vi "dryRunTest.vi"() -> ()   [LabVIEW 2015]
uses:
  GlobalPath.vi
  GlobalData.vi
  GlobalVi.vi
panel:
  in  "Done?":bool
  in  "Open Gauge Program 2":bool
  in  "Full or empty?":bool
  in  "Done?":bool
  in  "Open Gauge Program":bool
  in  "c-ccd 14":bool caption="Stiffback surface measurement with gauge system"
  in  "c-ccd 13":bool caption="Micrometer measurement of the distance between the reference plates \nand the stiffback plates along the perimeter"
  in  "c-ccd 12":bool caption="Position the weights on the stiffback"
  in  "c-ccd 11":bool caption="Release the stiffback from the movement arch"
  in  "c-ccd 10":bool caption="Lower the stiffback on the reference plates"
  in  "c-ccd 9":bool caption="Move the stiffback over the reference plates"
  in  "c-ccd 8":bool caption="Rotate the stiffback upside down"
  in  "c-ccd 7":bool caption="Check cleanness of the 20 stiffback supports"
  in  "c-ccd 6":bool caption="Mount the 2 stiffback-alignment pins on the reference plates"
  in  "c-ccd 5":bool caption="Position the honeycomb on the PCBs"
  in  "c-ccd 4":bool caption="Position the 4 internal frames in correspondence to the PCB-to-PCB junction"
  in  "c-ccd 3":bool caption="Position the 6 extrenal frames using 12 PTFE pins"
  # "Dry run preparation"
  # "Dry run empty/full"
  # "(True if full)"
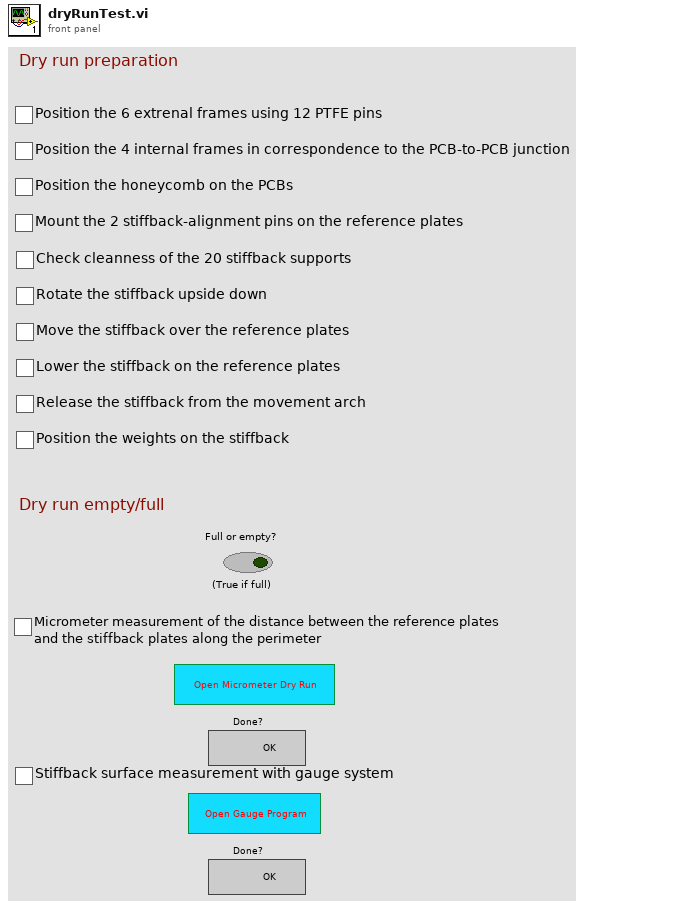
[diagram p1: front panel]
types:
  T1 = enum32{"Bad", "Idle", "Run top level", "Running"}
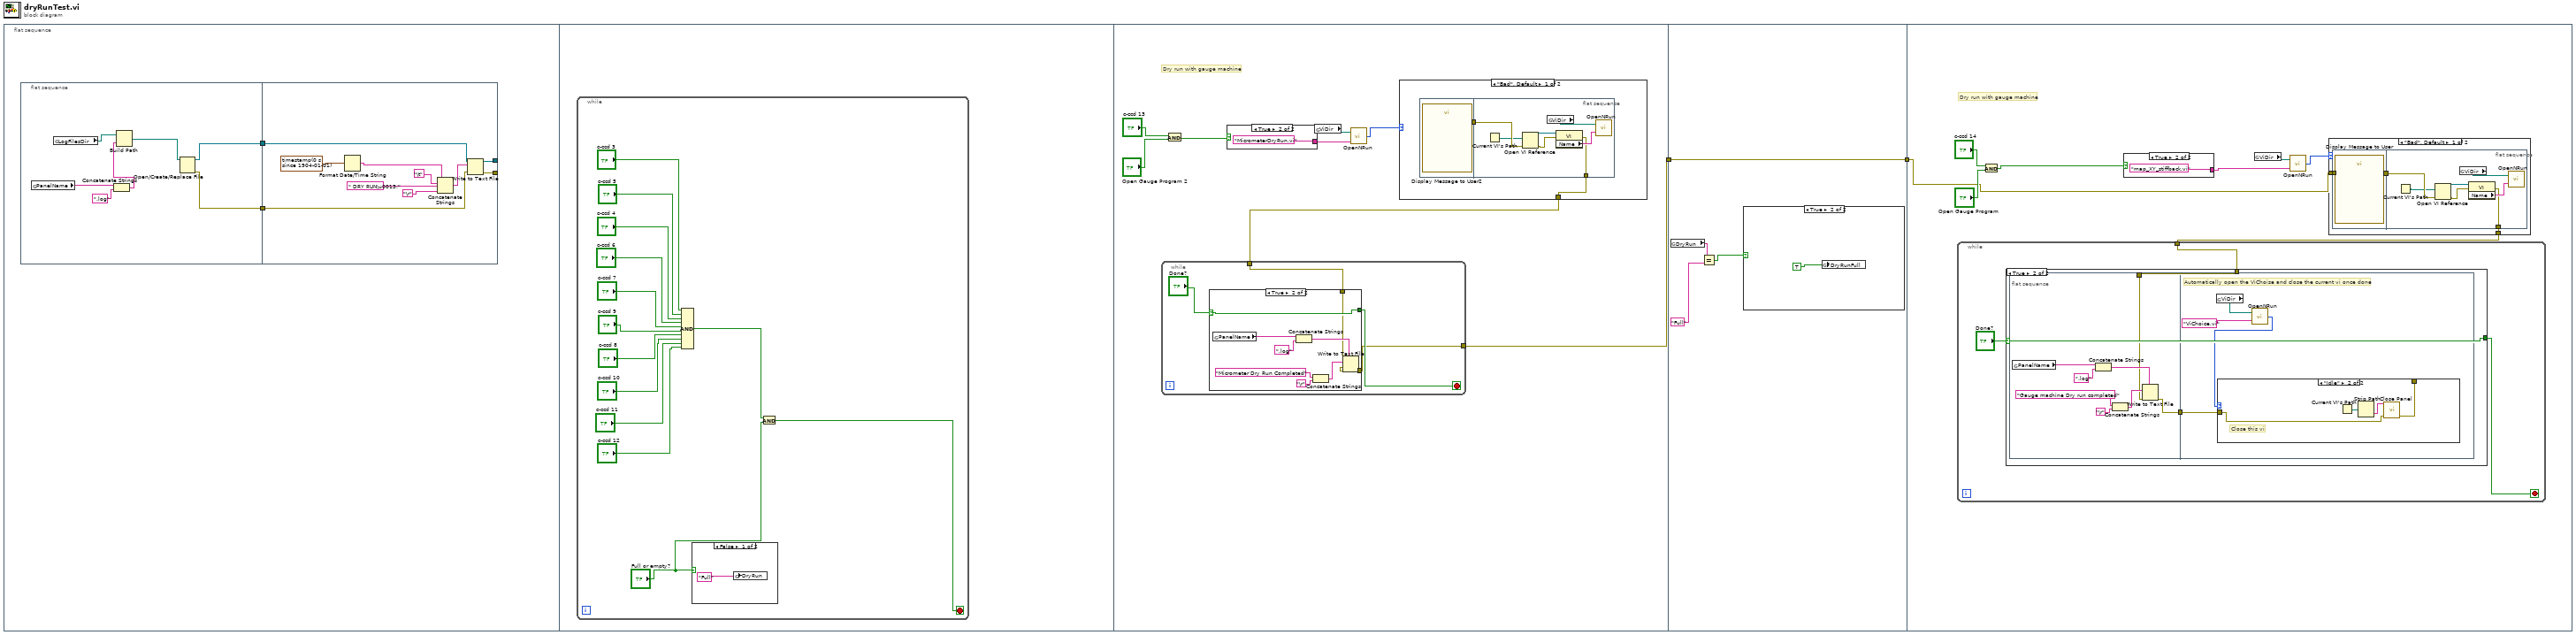
[diagram p0: block diagram]
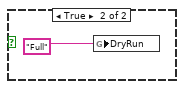
[diagram p2: hidden frame]
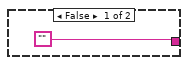
[diagram p5: hidden frame]
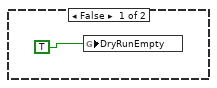
[diagram p6: hidden frame]
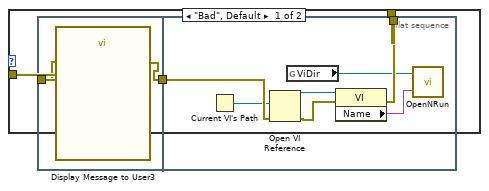
[diagram p8: hidden frame]
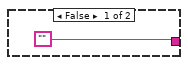
[diagram p10: hidden frame]
diagram:
  n1 = flat-sequence {
    tunnel: [w37] -> w2
    tunnel: w2 -> [w75]
    tunnel: [w75] -> w1
    tunnel: w1 -> [w78]
    frame #0 {
      n2 = flat-sequence {
        tunnel: [w6] -> w4
        tunnel: [w5] -> w3
        tunnel: w4 -> [w15]
        tunnel: [w14] -> _
        tunnel: [w13] -> _
        tunnel: w3 -> [w12]
        frame #0 {
          n3 = global read "GlobalData.vi" "PanelName"() -> (w9:string)
          n4 = global read "GlobalPath.vi" "LogFilesDir"() -> (w11:path)
          n5 = Concatenate Strings(w9, ".log") -> (w8:string)
          n6 = Build Path(base path=w11, name or relative path=w8) -> (appended path=w7:path)
          n7 = Open/Create/Replace File(file path (use dialog)=w7) -> (refnum out=w6:refnum<file>, error out=w5:errorcluster)  [unwired: 5 in, 1 out]
        }
        frame #1 {
          n8 = Format Date/Time String(seconds (now)=timestamp(0 s since 1904-01-01)) -> (date/time string=w18:string)  [unwired: 2 in]
          n9 = Concatenate Strings(w18, "\t", " DRY RUN\u0013:", "\r") -> (w16:string)
          n10 = Write to Text File(file (use dialog)=w15, text=w16, error in=w12) -> (refnum out=w14:refnum<file>, error out=w13:errorcluster)  [unwired: 1 in, 1 out]
        }
      }
    }
    frame #1 {
      n11 = while {
        stop <- w22 stop-if-true
        n12 = Compound Arithmetic op=AND("c-ccd 3", "c-ccd 5", "c-ccd 4", "c-ccd 6", "c-ccd 7", "c-ccd 9", "c-ccd 8", "c-ccd 10", "c-ccd 11", "c-ccd 12") -> (w23:bool)
        n13 = case shown="False" "Full or empty?" {
          frame False {
            n14 = global write "GlobalData.vi" "DryRun"("Full") -> ()
          }
          frame True {
            n15 = global write "GlobalData.vi" "DryRun"("Full") -> ()
          }
        }
        n16 = And(x=w23, y="Full or empty?") -> (x .and. y?=w22:bool)
      }
    }
    frame #2 {
      # "Dry run with gauge machine"
      n17 = And(x="c-ccd 13", y="Open Gauge Program 2") -> (x .and. y?=w40:bool)
      n18 = case shown="True" w40 {
        tunnel: ["" "MicrometerDryRun.vi"] -> w42
        frame False {
        }
        frame True {
        }
      }
      n19 = global read "GlobalPath.vi" "ViDir"() -> (w44:path)
      n20 = call "OpenNRun.vi"("VI name"=w42, "ViDirPath"=w44) -> ("Execution:State"=w43:T1)
      n21 = case shown="\"Bad\", Default" w43 {
        tunnel: [w60 _] -> w38
        frame "Bad", Default {
          n22 = flat-sequence {
            tunnel: [w62] -> w61
            tunnel: w61 -> [w65]
            tunnel: [w64] -> w60
            frame #0 {
              n23 = call "Display Message to User2"() -> ("error out"=w62:errorcluster)  [unwired: 10 in, 1 out]
            }
            frame #1 {
              n24 = Current VI's Path() -> (path=w63:path)
              n25 = Open VI Reference(vi path=w63, error in (no error)=w65) -> (vi reference=w69:refnum<vi>, error out=w68:errorcluster)  [unwired: 4 in]
              n26 = global read "GlobalPath.vi" "ViDir"() -> (w67:path)
              n27 = property class="VI"(reference=w69, error in=w68) -> (error out=w64:errorcluster, "Name"=w66:string)  [unwired: 1 out]
              n28 = call "OpenNRun.vi"("VI name"=w66, "ViDirPath"=w67) -> ()  [unwired: 1 out]
            }
          }
        }
        frame "Idle" {
        }
      }
      n29 = while {
        tunnel: w38 -> [w46]
        tunnel: [w45] -> w37
        stop <- w48 stop-if-true
        n30 = case shown="True" "Done?" {
          selector: "Done?" -> [w50 w53]
          tunnel: [w50 w53] -> w48
          tunnel: w46 -> [w49 w52]
          tunnel: [w49 w51] -> w45
          frame False {
          }
          frame True {
            n31 = global read "GlobalData.vi" "PanelName"() -> (w55:string)
            n32 = Concatenate Strings(w55, ".log") -> (w56:string)
            n33 = Concatenate Strings("Micrometer Dry Run Completed", "\r") -> (w59:string)
            n34 = Write to Text File(prompt (Choose or enter file path)=w56, text=w59, error in=w52) -> (error out=w51:errorcluster)  [unwired: 1 in, 2 out]
          }
        }
      }
    }
    frame #3 {
      n35 = global read "GlobalData.vi" "DryRun"() -> (w74:string)
      n36 = Equal?(x=w74, y="Full") -> (x = y?=w72:bool)
      n37 = case shown="True" w72 {
        frame False {
          n38 = global write "GlobalVi.vi" "DryRunEmpty"(TRUE) -> ()
        }
        frame True {
          n39 = global write "GlobalVi.vi" "DryRunFull"(TRUE) -> ()
        }
      }
    }
    frame #4 {
      # "Dry run with gauge machine"
      n40 = And(x="c-ccd 14", y="Open Gauge Program") -> (x .and. y?=w80:bool)
      n41 = case shown="True" w80 {
        tunnel: ["" "map_XY_stiffback.vi"] -> w83
        frame False {
        }
        frame True {
        }
      }
      n42 = global read "GlobalPath.vi" "ViDir"() -> (w85:path)
      n43 = call "OpenNRun.vi"("VI name"=w83, "ViDirPath"=w85) -> ("Execution:State"=w84:T1)
      n44 = case shown="\"Bad\", Default" w84 {
        tunnel: [w122 w133] -> w79
        tunnel: w78 -> [w121 w133]
        frame "Bad", Default {
          n45 = flat-sequence {
            tunnel: [w124] -> w123
            tunnel: w121 -> [w125]
            tunnel: w123 -> [w128]
            tunnel: [w127] -> w122
            frame #0 {
              n46 = call "Display Message to User"("error in (no error)"=w125) -> ("error out"=w124:errorcluster)  [unwired: 9 in, 1 out]
            }
            frame #1 {
              n47 = Current VI's Path() -> (path=w126:path)
              n48 = Open VI Reference(vi path=w126, error in (no error)=w128) -> (vi reference=w132:refnum<vi>, error out=w131:errorcluster)  [unwired: 4 in]
              n49 = global read "GlobalPath.vi" "ViDir"() -> (w130:path)
              n50 = property class="VI"(reference=w132, error in=w131) -> (error out=w127:errorcluster, "Name"=w129:string)  [unwired: 1 out]
              n51 = call "OpenNRun.vi"("VI name"=w129, "ViDirPath"=w130) -> ()  [unwired: 1 out]
            }
          }
        }
        frame "Idle" {
        }
      }
      n52 = while {
        tunnel: w79 -> [w86]
        stop <- w88 stop-if-true
        n53 = case shown="True" "Done?" {
          selector: "Done?" -> [w89 w90]
          tunnel: [w89 w90] -> w88
          tunnel: w86 -> [_ w92]
          frame False {
          }
          frame True {
            n54 = flat-sequence {
              tunnel: w92 -> [w94]
              tunnel: [w93] -> w91
              tunnel: w91 -> [w101]
              frame #0 {
                n55 = global read "GlobalData.vi" "PanelName"() -> (w96:string)
                n56 = Concatenate Strings(w96, ".log") -> (w97:string)
                n57 = Concatenate Strings("Gauge machine Dry run completed", "\r") -> (w100:string)
                n58 = Write to Text File(prompt (Choose or enter file path)=w97, text=w100, error in=w94) -> (error out=w93:errorcluster)  [unwired: 1 in, 2 out]
              }
              frame #1 {
                # "Automatically open the ViChoise and close the current vi once done"
                n59 = global read "GlobalPath.vi" "ViDir"() -> (w104:path)
                n60 = call "OpenNRun.vi"("VI name"="ViChoice.vi", "ViDirPath"=w104) -> ("Execution:State"=w103:T1)
                n61 = case shown="\"Idle\"" w103 {
                  tunnel: [w107 w117] -> _
                  tunnel: w101 -> [w106 w118]
                  frame "Bad", Default {
                    n62 = flat-sequence {
                      tunnel: w106 -> [w109]
                      tunnel: [w108] -> w105
                      tunnel: [w113] -> w107
                      tunnel: w105 -> [w112]
                      frame #0 {
                        n63 = call "Display Message to User3"("error in (no error)"=w109) -> ("error out"=w108:errorcluster)  [unwired: 9 in, 1 out]
                      }
                      frame #1 {
                        n64 = Current VI's Path() -> (path=w110:path)
                        n65 = Open VI Reference(vi path=w110, error in (no error)=w112) -> (vi reference=w116:refnum<vi>, error out=w115:errorcluster)  [unwired: 4 in]
                        n66 = global read "GlobalPath.vi" "ViDir"() -> (w111:path)
                        n67 = property class="VI"(reference=w116, error in=w115) -> (error out=w113:errorcluster, "Name"=w114:string)  [unwired: 1 out]
                        n68 = call "OpenNRun.vi"("VI name"=w114, "ViDirPath"=w111) -> ()  [unwired: 1 out]
                      }
                    }
                  }
                  frame "Idle" {
                    # "Close this vi"
                    n69 = Current VI's Path() -> (path=w120:path)
                    n70 = Strip Path(path=w120) -> (name=w119:string)  [unwired: 1 out]
                    n71 = call <vilib>:"Close Panel.vi"("error in (no error)"=w118, "VI name"=w119) -> ("error out"=w117:errorcluster)  [unwired: 9 in]
                  }
                }
              }
            }
          }
        }
      }
    }
  }
